vi "ImageAveragingFramesPointScan.vi"(6 "new":dbl[](array[numeric]), 7 "Frames grabbed":i32, 9 "Images 1D in":dbl[][](array[numeric]), 10 "y-index":i32, 11 "Image in":refnum<class "Image.lvclass">) -> (3 "Images 2D out":dbl[][](array[numeric]))   [LabVIEW 2012, in "Image.lvclass"]
uses:
  classes/Image.lvclass
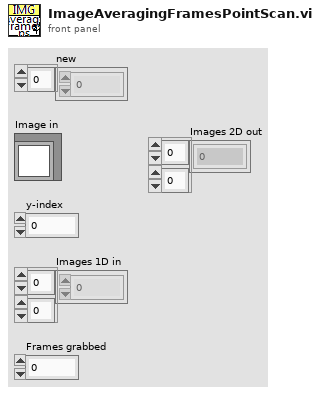
[diagram p1: front panel]
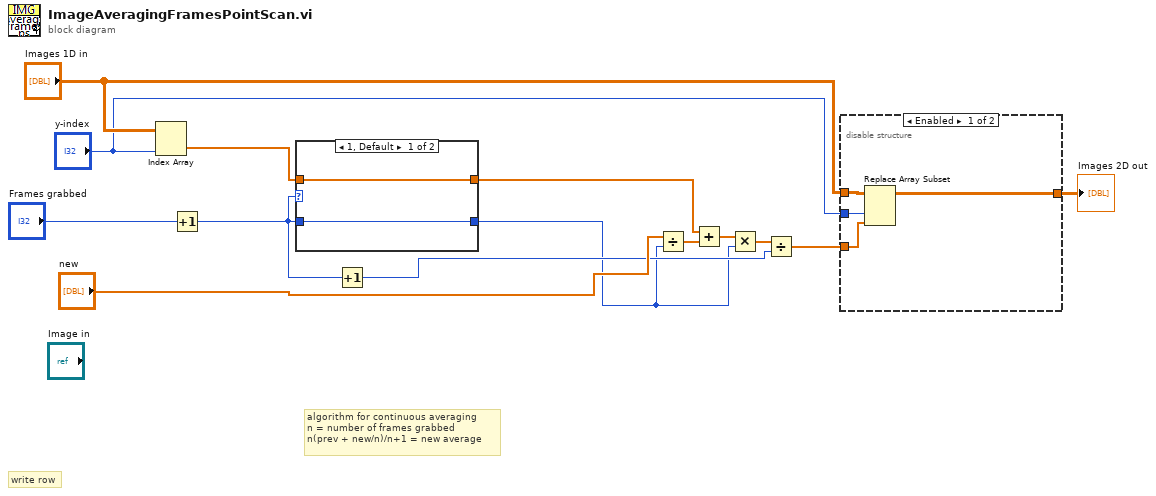
[diagram p0: block diagram]
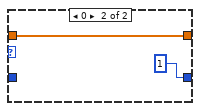
[diagram p2: hidden frame]
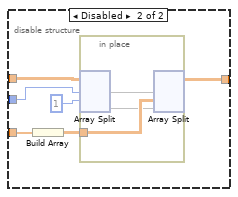
[diagram p3: hidden frame]
diagram:
  # "algorithm for continuous averaging\nn = number of frames grabbed\nn(prev + new/n)/n+1 = new average"
  # "write row"
  n1 = Index Array(array="Images 1D in", index (col)="y-index") -> (element=w13:dbl[])  [unwired: 1 in]
  n2 = Increment(x="Frames grabbed") -> (x+1=w9:i32)
  n3 = case shown="1, Default" w9 {
    tunnel: w9 -> [w16 _]
    tunnel: [w16 1 ("Frames grabbed")] -> w4
    tunnel: [w15 w17] -> w1
    tunnel: w13 -> [w15 w17]
    frame 1, Default {
    }
    frame 0 {
    }
  }
  n4 = Increment(x=w9) -> (x+1=w6:i32)
  n5 = Divide(x="new", y=w4) -> (x/y=w2:dbl[])
  n6 = Add(x=w1, y=w2) -> (x+y=w5:dbl[])
  n7 = Multiply(x=w5, y=w4) -> (x*y=w3:dbl[])
  n8 = Divide(x=w3, y=w6) -> (x/y=w12:dbl[])
  n9 = disable-structure shown="Enabled" {
    disable-tunnel: w12 -> [w22 w25]
    disable-tunnel: [w21 w23] -> w11
    disable-tunnel: "Images 1D in" -> [w20 w28]
    disable-tunnel: "y-index" -> [w19 w26]
    frame Enabled {
      n10 = Replace Array Subset(array=w20, new element=w22, index (col)=w19) -> (w21:dbl[][])  [unwired: 1 in]
    }
    frame Disabled {
      n11 = Build Array(w25) -> (w24:dbl[][])
      n12 = in-place {
        in-place-border: w24 -> [w30]
        n13 = in-place-split #1(w28, w26, 1) -> (w31:dbl[][], w29:dbl[][])  [unwired: 1 out]
        n14 = in-place-split #1(w31, w30, w29) -> (w23:dbl[][])  [unwired: 2 out]
      }
    }
  }
  "Images 2D out" <- w11
